vi "纳清DO_所有参数读取.vi"(5 "大气压补偿":dbl, 7 "盐度补偿":dbl, 8 "error in (no error)":errorcluster caption="错误输入（无错误）", 11 "MB session in":refnum<class "MB_Master.lvclass">) -> (0 "error out":errorcluster caption="错误输出", 2 "输出值":T1 {"波特率" items=["4800", "9600", "19200", "38400", "57600", "115200"]}, 3 "MB session out":refnum<class "MB_Master.lvclass">)   [LabVIEW 2016, in "斯坦道多参数.lvlib"]
uses:
  <vilib>/Plasmionique/MB Master/MB_Master/MB_Master.lvclass
  <vilib>/Plasmionique/MB Master/MB Master.lvlib
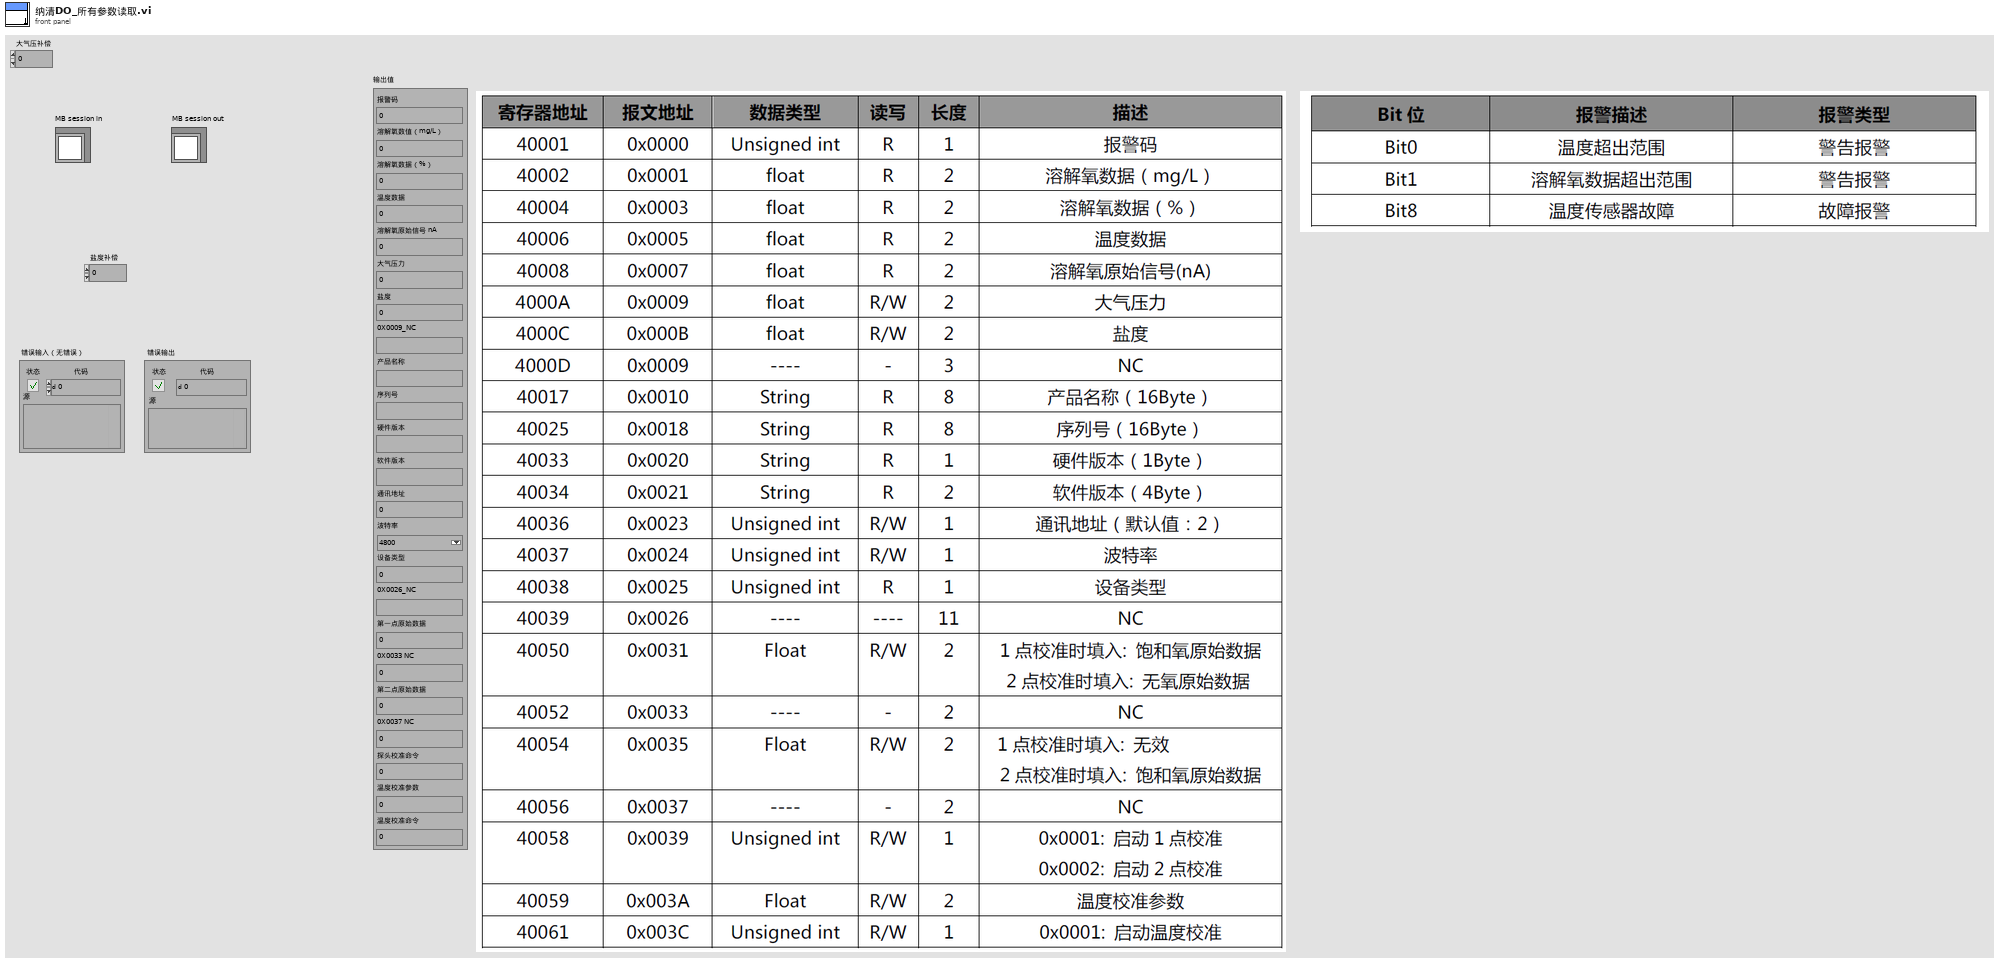
[diagram p1: front panel]
types:
  T1 = cluster{"报警码":u16, "溶解氧数值（mg/L）":sgl, "溶解氧数据（%）":sgl, "温度数据":sgl, "溶解氧原始信号 nA":sgl, "大气压力":sgl, "盐度":sgl, "0X0009_NC":string, "产品名称":string, "序列号":string, "硬件版本":string, "软件版本":string, "通讯地址":u16, "波特率":u16, "设备类型":u16, "0X0026_NC":string, "第一点原始数据":sgl, "0X0033 NC":sgl, "第二点原始数据":sgl, "0X0037 NC":sgl, "探头校准命令":u16, "温度校准参数":sgl, "温度校准命令":u16}
  T2 = cluster{"pH":u32, "DO":u32, "Cond":u32, "Turb":u32, "叶绿素a":u32, "藻密度":u32, "ORP":u32, "COD":u32, "氯化物":u32, "氨氮":u32, "水中油":u32, "悬浮物":u32, "余氯":u32}
  T3 = cluster{u16, "mode":dbl, "数值":sgl, "数值":sgl, "数值":sgl, "大气压补偿":dbl, "盐度补偿":dbl, "类型":string, "类型":string, "类型":string, "类型":string, "类型":string, u16, u16, u16, "类型":string, "数值":sgl, "数值":sgl, "数值":sgl, "数值":sgl, u16, "数值":sgl, u16}
  T4 = cluster{"报警码":u16, "溶解氧数值（mg/L）":sgl, "溶解氧数据（%）":sgl, "温度数据":sgl, "溶解氧原始信号 nA":sgl, "大气压力":sgl, "盐度":sgl, "0X0009_NC":string, "产品名称":string, "序列号":string, "硬件版本":string, "软件版本":string, "通讯地址":u16, "波特率":u16, "设备类型":u16, "0X0026_NC":string, "第一点原始数据":sgl, "第一点校准数据":sgl, "第二点原始数据":sgl, "第二点校准数据":sgl, "探头校准命令":u16, "温度校准参数":sgl, "温度校准命令":u16}
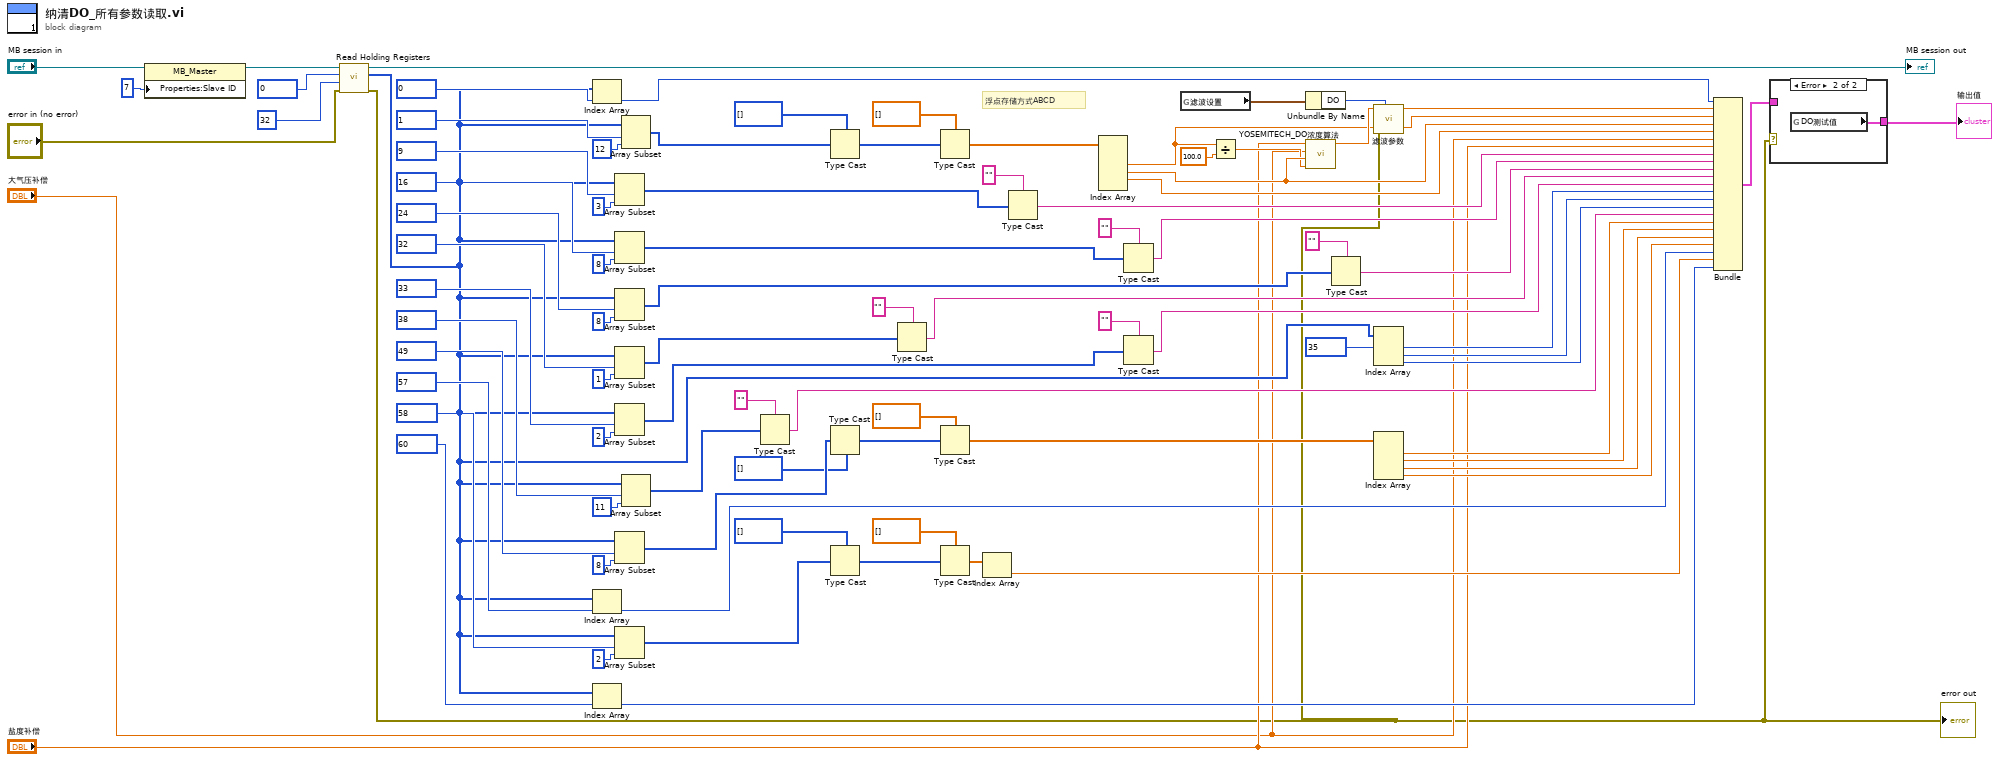
[diagram p0: block diagram]
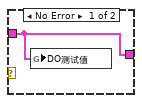
[diagram p2: hidden frame]
diagram:
  # "浮点存储方式ABCD"
  n1 = property class="MB_Master"(reference="MB session in", "Properties:Slave ID"=u8 7 ("Slave ID")) -> (reference out=w78:refnum<class "MB_Master.lvclass">)  [unwired: 1 in, 1 out]
  n2 = call <vilib>:"Read Holding Registers.vi"("error in (no error)"="error in (no error)", "quantity"=u16 32, "starting address"=u16 0, "MB session in"=w78) -> ("error out"=w1:errorcluster, "Registers"=w22:u16[], "MB session out"=→"MB session out":refnum<class "MB_Master.lvclass">)  [unwired: 5 in]
  "error out" <- w1
  n3 = Index Array(array=w22, index=u16 0 ("starting address")) -> (element=w86:u16)
  n4 = Index Array(array=w22, index=u16 57 ("starting address")) -> (element=w25:u16)
  n5 = Index Array(array=w22, index=u16 60 ("starting address")) -> (element=w21:u16)
  n6 = Array Subset(array=w22, index=u16 9 ("starting address"), length=3 ("长度")) -> (w73:u16[])
  n7 = Array Subset(array=w22, index=u16 16 ("starting address"), length=8 ("长度")) -> (w69:u16[])
  n8 = Array Subset(array=w22, index=u16 24 ("starting address"), length=8 ("长度")) -> (w63:u16[])
  n9 = Array Subset(array=w22, index=u16 32 ("starting address"), length=1 ("长度")) -> (w59:u16[])
  n10 = Array Subset(array=w22, index=u16 33 ("starting address"), length=2 ("长度")) -> (w53:u16[])
  n11 = Array Subset(array=w22, index=u16 49 ("starting address"), length=8 ("长度")) -> (w40:u16[])
  n12 = Array Subset(array=w22, index=u16 58 ("starting address"), length=2 ("长度")) -> (w28:u16[])
  n13 = Array Subset(array=w22, index=u16 1 ("starting address"), length=12 ("长度")) -> (w82:u16[])
  n14 = Array Subset(array=w22, index=u16 38 ("starting address"), length=11 ("长度")) -> (w43:u16[])
  n15 = Type Cast(type="" ("类型"), x=w43) -> (*(type *) &x=w42:string)
  n16 = Type Cast(type=u32[] [] ("数组 2"), x=w82) -> (*(type *) &x=w20:u32[])
  n17 = Type Cast(type=u32[] [] ("数组 2"), x=w40) -> (*(type *) &x=w38:u32[])
  n18 = Type Cast(type=u32[] [] ("数组 2"), x=w28) -> (*(type *) &x=w30:u32[])
  n19 = Type Cast(type="" ("类型"), x=w59) -> (*(type *) &x=w56:string)
  n20 = Type Cast(type=sgl[] [] ("数组 2"), x=w20) -> (*(type *) &x=w81:sgl[])
  n21 = Type Cast(type=sgl[] [] ("数组 2"), x=w38) -> (*(type *) &x=w35:sgl[])
  n22 = Type Cast(type=sgl[] [] ("数组 2"), x=w30) -> (*(type *) &x=w33:sgl[])
  n23 = Index Array(array=w33) -> (element=w24:sgl)  [unwired: 1 in]
  n24 = Type Cast(type="" ("类型"), x=w73) -> (*(type *) &x=w71:string)
  n25 = Index Array(array=w81) -> (element #2=w7:sgl, element #3=w9:sgl, element #4=w17:sgl)  [unwired: 5 in, 2 out]
  n26 = Type Cast(type="" ("类型"), x=w69) -> (*(type *) &x=w66:string)
  n27 = Type Cast(type="" ("类型"), x=w53) -> (*(type *) &x=w51:string)
  n28 = global read "断电保存变量.vi" "滤波设置"() -> (w11:T2)
  n29 = Divide(x=w7, y=sgl 100.0) -> (x/y=w5:sgl)
  n30 = Unbundle By Name(w11) -> ("DO"=w10:u32)
  n31 = call "YOSEMITECH_DO浓度算法.vi"("溶解氧饱和度值"=w5, "水温"=w9, "大气压补偿"="大气压补偿", "盐度补偿"="盐度补偿") -> ("DataDo_mgL"=w8:dbl)  [unwired: 7 in]
  n32 = Type Cast(type="" ("类型"), x=w63) -> (*(type *) &x=w61:string)
  n33 = call "滤波参数.vi"("滤波次数"=w10, "error in (no error)"=w1, "x"=w8) -> ("mode"=w12:dbl)  [unwired: 7 in, 1 out]
  n34 = Index Array(array=w22, index #1=u16 35 ("starting address")) -> (element #1=w49:u16, element #2=w48:u16, element #3=w47:u16)  [unwired: 2 in]
  n35 = Index Array(array=w35) -> (element #1=w34:sgl, element #2=w16:sgl, element #3=w15:sgl, element #4=w14:sgl)  [unwired: 4 in]
  n36 = Bundle(w86, "mode"=w12, "数值"=w7, "数值"=w9, "数值"=w17, "大气压补偿"="大气压补偿", "盐度补偿"="盐度补偿", "类型"=w71, "类型"=w66, "类型"=w61, "类型"=w56, "类型"=w51, w49, w48, w47, "类型"=w42, "数值"=w34, "数值"=w16, "数值"=w15, "数值"=w14, w25, "数值"=w24, w21) -> (w13:T3)  [unwired: 1 in]
  n37 = case shown="Error" w1 {
    tunnel: w13 -> [w89 _]
    tunnel: [w89 w90] -> w3
    frame No Error {
      n38 = global write "纳清过程全局变量.vi" "DO测试值"(w89) -> ()
    }
    frame Error {
      n39 = global read "纳清过程全局变量.vi" "DO测试值"() -> (w90:T4)
    }
  }
  "输出值" <- w3
